vi "convertFITS.vi"(8 "error in (no error)":errorcluster, 10 "Header data cluster":T1, 11 "Input CSV File path":path) -> (0 "error out":errorcluster, 2 "Success?":bool, 3 "Out Fits File":path)   [LabVIEW 2019]
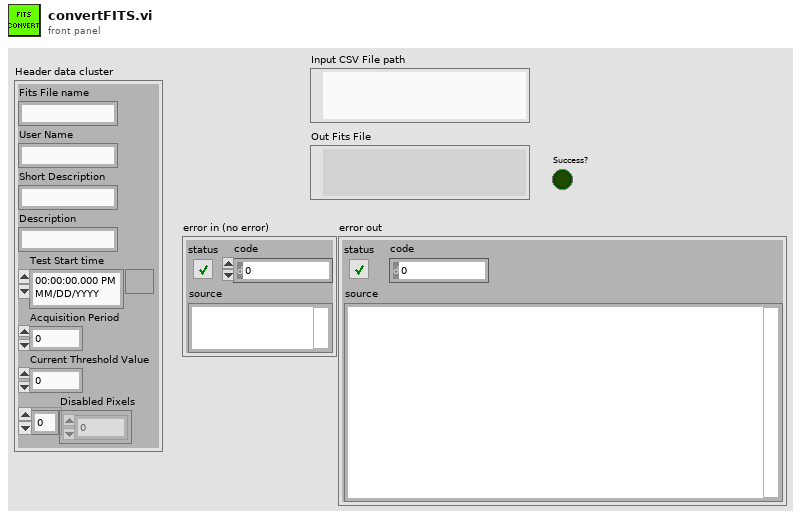
[diagram p1: front panel]
types:
  T1 = cluster{"Fits File name":string, "User Name":string, "Short Description":string, "Description":string, "Test Start time":timestamp, "Acquisition Period":dbl, "Current Threshold Value":u16, "Disabled Pixels":u8[]}
  T2 = cluster{"Fits File Name":string, "Fits File Path":string, "User Name":string, "Short Description":string, "Test Start Time":string, "Acquisition Period":string, "Energy Threshold":string, "Disabled Pixels":string, "Description":string}
  T3 = enum32{"invalid app kind", "Development System", "Run Time System", "Student Edition", "Embedded LabVIEW", "Evaluation", "Custom"}
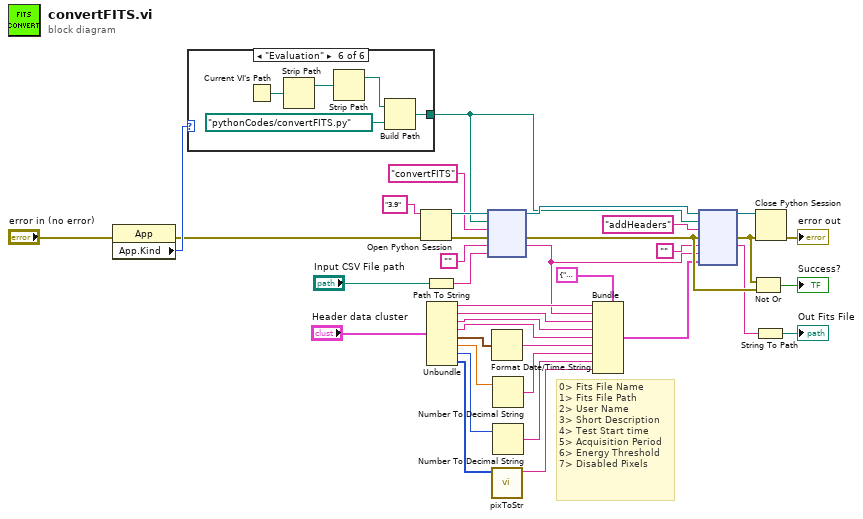
[diagram p0: block diagram]
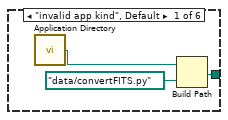
[diagram p2: hidden frame]
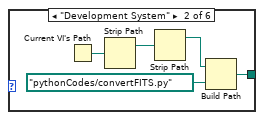
[diagram p3: hidden frame]
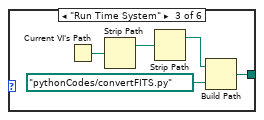
[diagram p4: hidden frame]
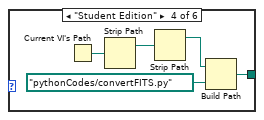
[diagram p5: hidden frame]
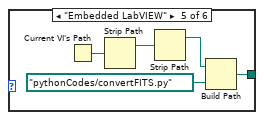
[diagram p6: hidden frame]
diagram:
  # "0> Fits File Name\n1> Fits File Path\n2> User Name\n3> Short Description\n4> Test Start time\n5> Acquisition Period\n6> Energy Threshold \n7> Disabled Pixels"
  n1 = property class="App"(error in="error in (no error)") -> (error out=w1:errorcluster, "App.Kind"=w3:T3)  [unwired: 1 in, 1 out]
  n2 = case shown="\"Evaluation\"" w3 {
    tunnel: [w38 w41 w46 w51 w56 w61] -> w5
    frame "invalid app kind", Default {
      n3 = call <vilib>:"Application Directory.vi"() -> ("Application Directory"=w39:path)
      n4 = Build Path(base path=w39, name or relative path=path "data/convertFITS.py" ("stripped path 2")) -> (appended path=w38:path)
    }
    frame "Development System" {
      n5 = Current VI's Path() -> (path=w45:path)
      n6 = Strip Path(path=w45) -> (stripped path=w44:path)  [unwired: 1 out]
      n7 = Strip Path(path=w44) -> (stripped path=w43:path)  [unwired: 1 out]
      n8 = Build Path(base path=w43, name or relative path=path "pythonCodes/convertFITS.py" ("stripped path 2")) -> (appended path=w41:path)
    }
    frame "Run Time System" {
      n9 = Current VI's Path() -> (path=w50:path)
      n10 = Strip Path(path=w50) -> (stripped path=w49:path)  [unwired: 1 out]
      n11 = Strip Path(path=w49) -> (stripped path=w48:path)  [unwired: 1 out]
      n12 = Build Path(base path=w48, name or relative path=path "pythonCodes/convertFITS.py" ("stripped path 2")) -> (appended path=w46:path)
    }
    frame "Student Edition" {
      n13 = Current VI's Path() -> (path=w55:path)
      n14 = Strip Path(path=w55) -> (stripped path=w54:path)  [unwired: 1 out]
      n15 = Strip Path(path=w54) -> (stripped path=w53:path)  [unwired: 1 out]
      n16 = Build Path(base path=w53, name or relative path=path "pythonCodes/convertFITS.py" ("stripped path 2")) -> (appended path=w51:path)
    }
    frame "Embedded LabVIEW" {
      n17 = Current VI's Path() -> (path=w60:path)
      n18 = Strip Path(path=w60) -> (stripped path=w59:path)  [unwired: 1 out]
      n19 = Strip Path(path=w59) -> (stripped path=w58:path)  [unwired: 1 out]
      n20 = Build Path(base path=w58, name or relative path=path "pythonCodes/convertFITS.py" ("stripped path 2")) -> (appended path=w56:path)
    }
    frame "Evaluation" {
      n21 = Current VI's Path() -> (path=w65:path)
      n22 = Strip Path(path=w65) -> (stripped path=w64:path)  [unwired: 1 out]
      n23 = Strip Path(path=w64) -> (stripped path=w63:path)  [unwired: 1 out]
      n24 = Build Path(base path=w63, name or relative path=path "pythonCodes/convertFITS.py" ("stripped path 2")) -> (appended path=w61:path)
    }
  }
  n25 = Open Python Session(python version="3.9", 3:w1) -> (session out=w37:refnum<k35>, error out=w36:errorcluster)  [unwired: 1 in]
  n26 = Path To String(path="Input CSV File path") -> (string=w27:string)
  n27 = Unbundle("Header data cluster") -> ("Fits File name"=w26:string, "User Name"=w25:string, "Short Description"=w24:string, "Description"=w8:string, "Test Start time"=w13:timestamp, "Acquisition Period"=w14:dbl, "Current Threshold Value"=w15:u16, "Disabled Pixels"=w16:u8[])
  n28 = node(w37, w5, "convertFITS", w36, "", w27) -> (w32:refnum<k35>, w21:errorcluster, w7:string)  [unwired: 1 in, 2 out]
  n29 = Format Date/Time String(seconds (now)=w13) -> (date/time string=w9:string)  [unwired: 2 in]
  n30 = call "pixToStr.vi"("Disabled Pixels"=w16) -> ("Disabled pixels string"=w12:string)  [unwired: 10 in]
  n31 = Number To Decimal String(number=w14) -> (decimal integer string=w10:string)  [unwired: 1 in]
  n32 = Number To Decimal String(number=w15) -> (decimal integer string=w11:string)  [unwired: 1 in]
  n33 = Bundle(cluster=T2 {"Fits File Name"="", "Fits File Path"="", "User Name"="", "Short Description"="", "Test Start Time"="", "Acquisition Period"="100", "Energy Threshold"="", "Disabled Pixels"="", "Description"=""}, "Fits File Name"=w26, "Fits File Path"=w7, "User Name"=w25, "Short Description"=w24, "Test Start Time"=w8, "Acquisition Period"=w9, "Energy Threshold"=w10, "Disabled Pixels"=w11, "Description"=w12) -> (w18:T2)
  n34 = node(w32, w5, "addHeaders", w21, "", w7, w18) -> (w31:refnum<k35>, w20:errorcluster, w6:string)  [unwired: 2 in, 2 out]
  n35 = Not Or(1:w21, 2:w20) -> (0:→"Success?":bool)
  n36 = String To Path(string=w6) -> (path=→"Out Fits File":path)
  n37 = Close Python Session(session in=w31, error in=w20) -> (11:→"error out":errorcluster)
